vi "PickDropVacCtrld.vi"(7 "VacuumState":u32=50331648, 8 "error in (no error)":errorcluster, 9 "controller in":refnum<k24>, 10 "Zspeed":dbl=50.0 format="%#_13g", 11 "Z":dbl=65.0) -> (0 "error out":errorcluster, 3 "controller out":refnum<k24>)   [LabVIEW 2021]
uses:
  C:/Users/TTUHEP/Documents/LabVIEW/Other Models/2010/Bin/Aerotech.A3200.dll
  Other Models/2010/Bin/Aerotech.A3200.dll
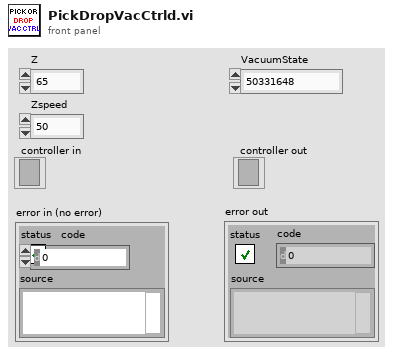
[diagram p1: front panel]
types:
  T1 = enum16{"Conversion", "BinarySwitch", "DecimalSwitch"}
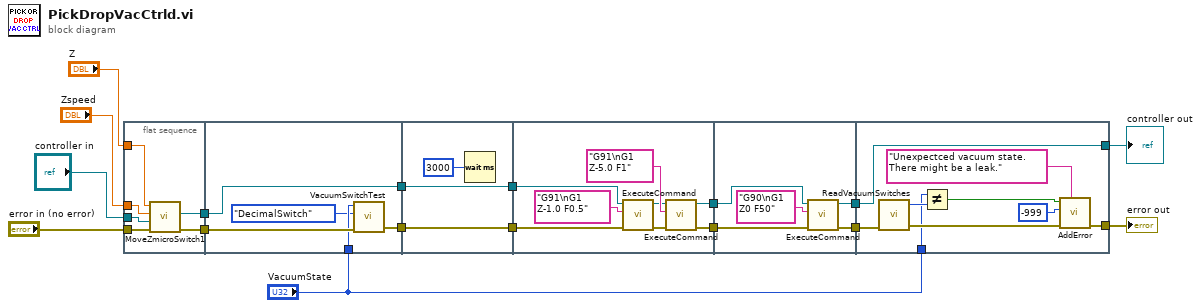
[diagram p0: block diagram]
diagram:
  n1 = flat-sequence {
    tunnel: [w20] -> w17
    tunnel: [w21] -> w16
    tunnel: "controller in" -> [w23]
    tunnel: "error in (no error)" -> [w22]
    tunnel: "Z" -> [w19]
    tunnel: "Zspeed" -> [w18]
    tunnel: w17 -> [w28]
    tunnel: [w26] -> w11
    tunnel: [w27] -> w10
    tunnel: w16 -> [w27]
    tunnel: "VacuumState" -> [w25]
    tunnel: w11 -> [w31]
    tunnel: [w31] -> w4
    tunnel: w10 -> [w30]
    tunnel: [w30] -> w2
    tunnel: w4 -> [w37]
    tunnel: [w32] -> w3
    tunnel: w2 -> [w38]
    tunnel: [w33] -> w1
    tunnel: w3 -> [w44]
    tunnel: w1 -> [w42]
    tunnel: [w41] -> w9
    tunnel: [w40] -> w8
    tunnel: w9 -> [w48]
    tunnel: w8 -> [w46]
    tunnel: [w47] -> w7
    tunnel: [w46] -> w6
    tunnel: "VacuumState" -> [w45]
    frame #0 {
      n2 = call "MoveZmicroSwitch1.vi"("Z"=w19, "Zspeed"=w18, "controller in"=w23, "error in (no error)"=w22) -> ("controller out"=w21:refnum<k24>, "error out"=w20:errorcluster)  [unwired: 3 in, 2 out]
    }
    frame #1 {
      n3 = call "VacuumSwitchTest.vi"("Error In"=w28, "ControlType"=T1."DecimalSwitch", "DecimalIn"=w25) -> ("error out"=w26:errorcluster)  [unwired: 1 in, 2 out]
    }
    frame #2 {
      n4 = Wait (ms)(milliseconds to wait=u32 3000) -> ()  [unwired: 1 out]
    }
    frame #3 {
      n5 = call "ExecuteCommand.vi"("error in (no error)"=w37, "Command Code"="G91\nG1 Z-1.0 F0.5", "controller in"=w38) -> ("error out"=w34:errorcluster, "controller out"=w35:refnum<k24>)  [unwired: 6 in, 1 out]
      n6 = call "ExecuteCommand.vi"("error in (no error)"=w34, "Command Code"="G91\nG1 Z-5.0 F1", "controller in"=w35) -> ("error out"=w32:errorcluster, "controller out"=w33:refnum<k24>)  [unwired: 6 in, 1 out]
    }
    frame #4 {
      n7 = call "ExecuteCommand.vi"("error in (no error)"=w44, "Command Code"="G90\nG1 Z0 F50", "controller in"=w42) -> ("error out"=w41:errorcluster, "controller out"=w40:refnum<k24>)  [unwired: 6 in, 1 out]
    }
    frame #5 {
      n8 = call "ReadVacuumSwitches.vi"("error in"=w48) -> ("OutVacStatus"=w51:u32, "error out"=w52:errorcluster)  [unwired: 4 in, 1 out]
      n9 = Not Equal?(x=w45, y=w51) -> (x != y?=w53:bool)
      n10 = call "AddError.vi"("ErrorMessage"="Unexpectced vacuum state. There might be a leak.", "error in"=w52, "code"=-999, "Error?"=w53) -> ("Error out"=w47:errorcluster)  [unwired: 7 in]
    }
  }
  "controller out" <- w6
  "error out" <- w7
